vi "Module Loop.vi"(8 "error in (no error)":errorcluster, 11 "GenericGuiAO in":refnum<class "GenericGuiDO.lvclass">) -> (0 "error out":errorcluster, 3 "GenericGuiAO out":refnum<class "GenericGuiDO.lvclass">)   [LabVIEW 2020, in "VolatusDAQGenericGUI.lvlib" / "GenericGuiDO.lvclass"]
uses:
  GenericGuiDO.lvclass
  C:/dev/lv20CE/relink/lv-volatus/Volatus/Module/Module.lvclass
  Volatus/Module/Module.lvclass/Module.ctl
  Volatus/MessageQ/MessageQ.lvclass/MessageQ.ctl
  Volatus/Module/Module.lvclass
  GenericGuiDO.lvclass/GenericGuiDO.ctl
  <vilib>/Utility/error.llb/Error Cluster From Error Code.vi
  Volatus/MessageQ/MessageQ.lvclass
  VolatusDAQGenericGUI.lvlib
  C:/dev/lv20CE/relink/lv-volatus/VolatusDAQGenericGUI/GenericGuiDO/GenericGuiDO.lvclass
  Volatus/VolatusAPI/VolatusAPI.lvclass
panel:
  in  "Tree":string(tree)
  out "Cover":string="\n\n\n\n\n\n\nSelect Channel to command"
  in  "Value":bool
  out "Channel":string
  in  "Send Command":bool
  in  "Live Command":bool
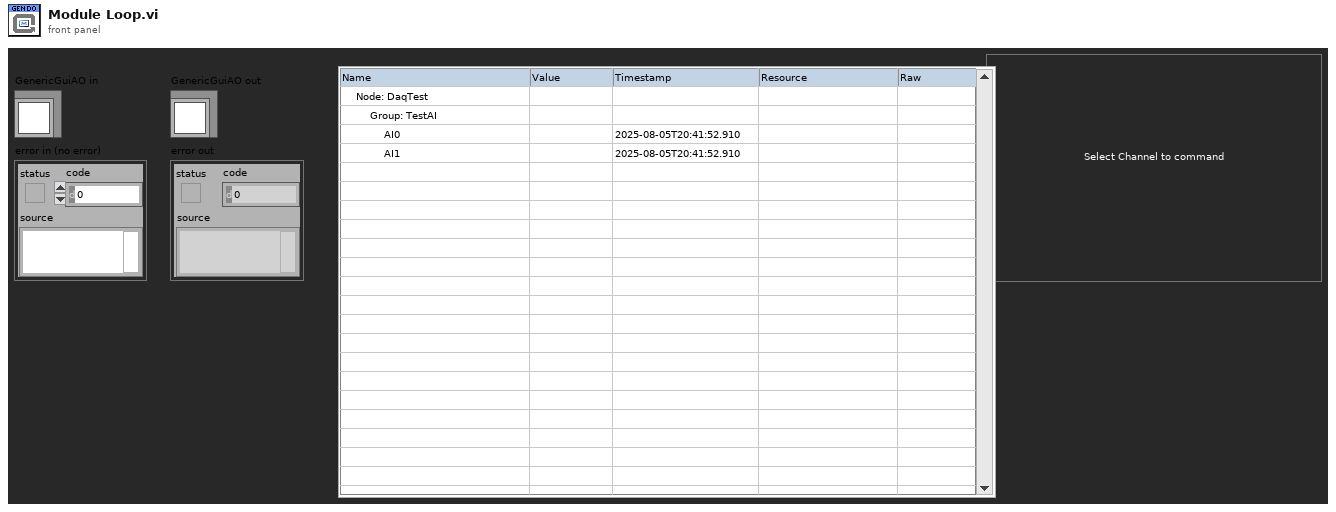
[diagram p1: front panel]
types:
  T1 = enum32{"Invalid", "Standard", "Closed", "Hidden", "Minimized", "Maximized"}
  T2 = typedef "VolatusDAQGenericGUI.lvlib/Group Info.ctl" = cluster{"Group":refnum<class "Group.lvclass">, "Channel Names":string[], "Resources":string[], "Node":string, "Task":string}
  T3 = enum8{"Enabled", "Disabled", "Disabled and Grayed Out"}
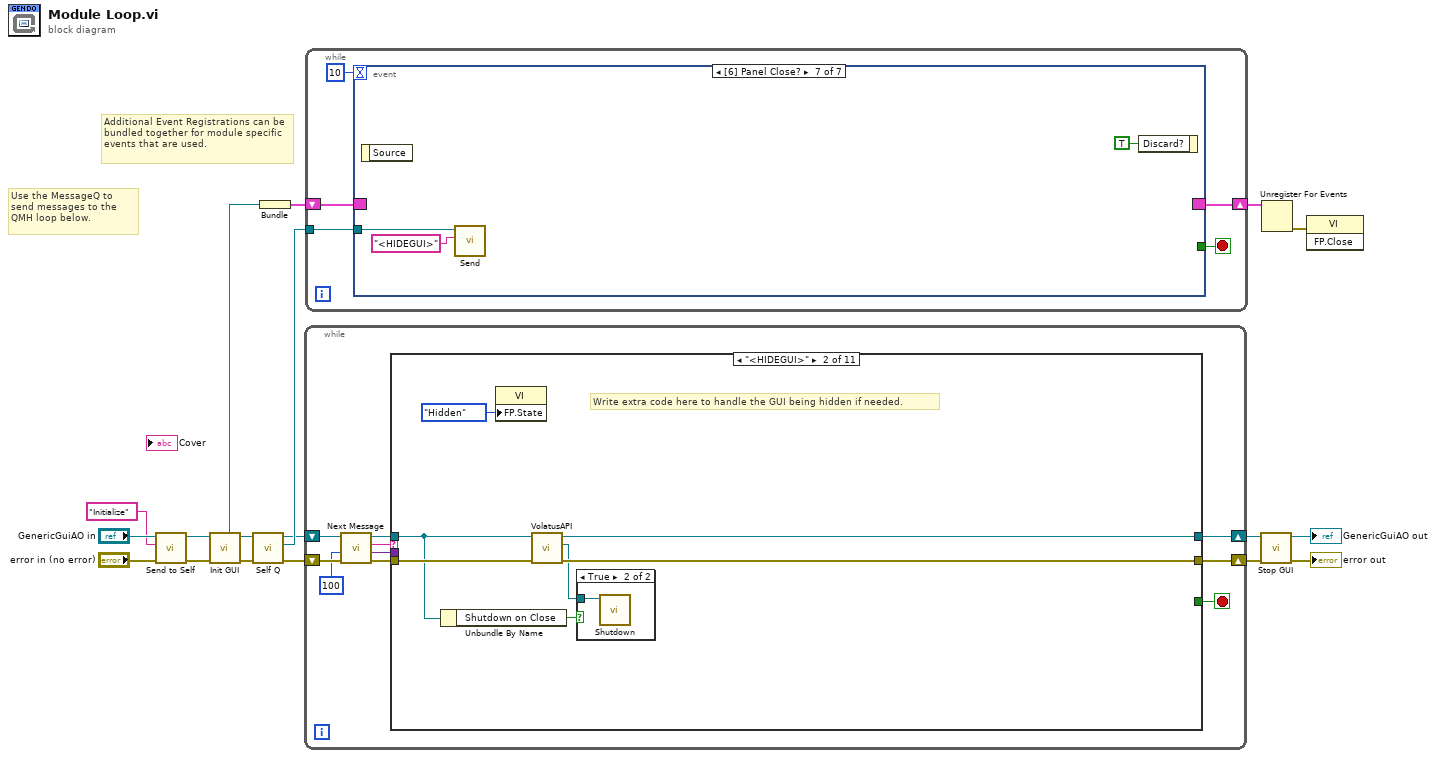
[diagram p0: block diagram]
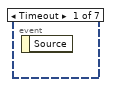
[diagram p2: hidden frame]
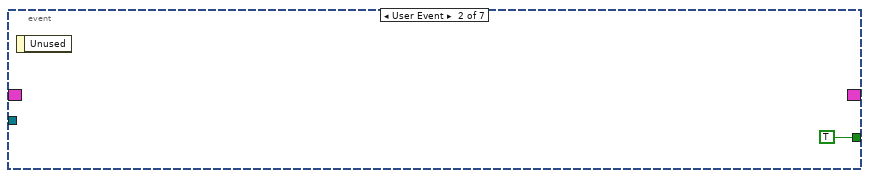
[diagram p3: hidden frame]
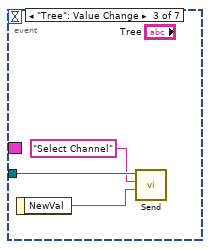
[diagram p4: hidden frame]
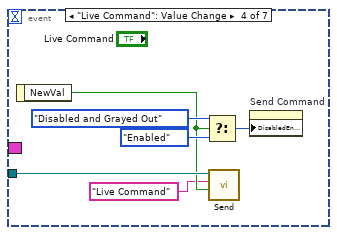
[diagram p5: hidden frame]
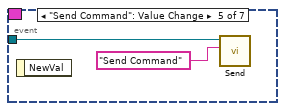
[diagram p6: hidden frame]
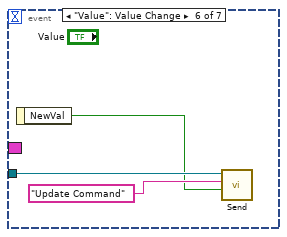
[diagram p7: hidden frame]
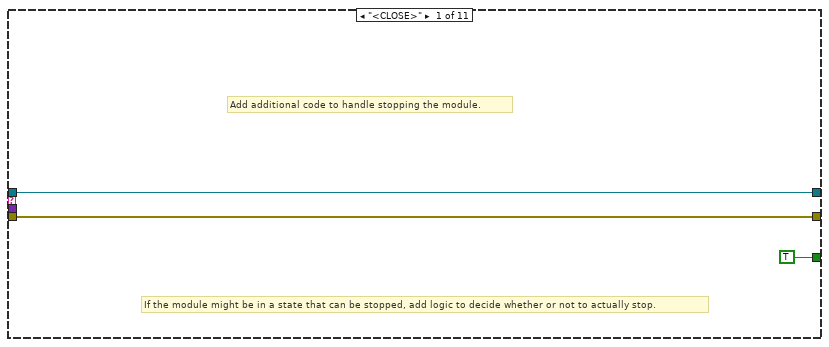
[diagram p8: hidden frame]
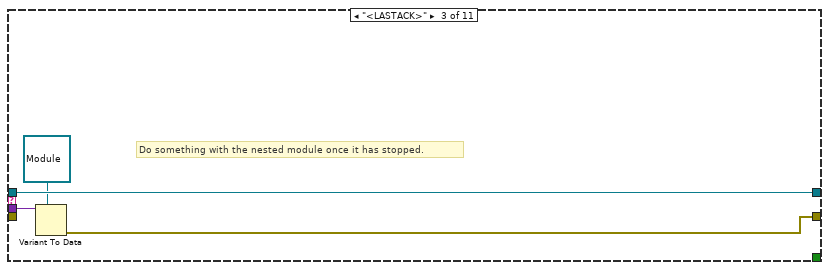
[diagram p10: hidden frame]
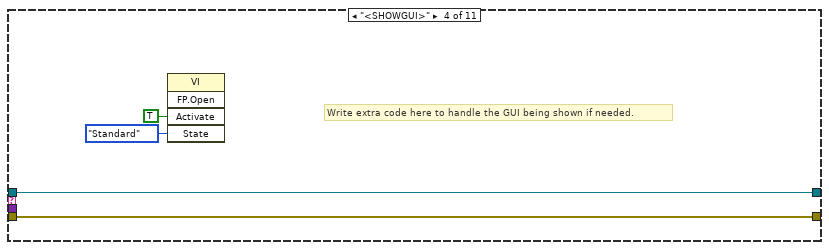
[diagram p11: hidden frame]
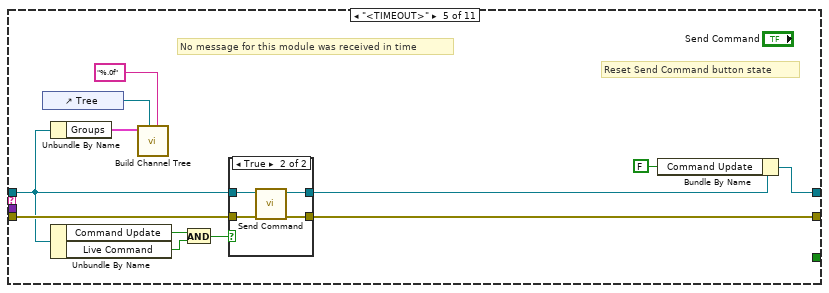
[diagram p12: hidden frame]
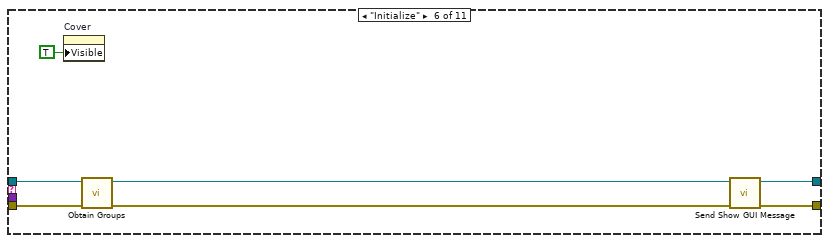
[diagram p14: hidden frame]
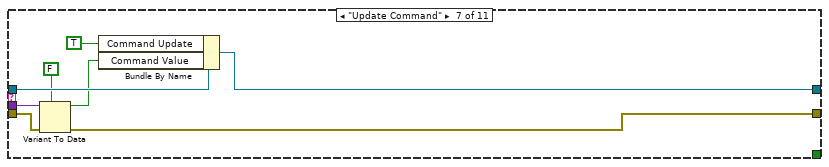
[diagram p15: hidden frame]
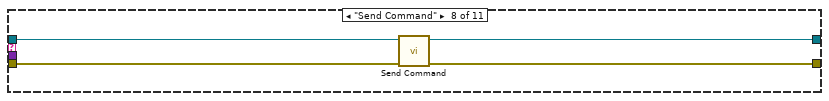
[diagram p16: hidden frame]
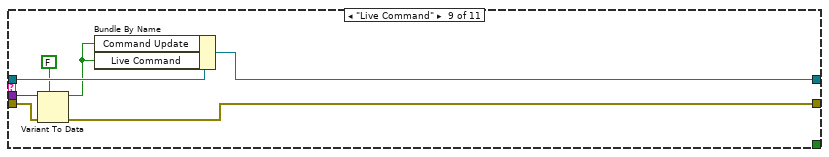
[diagram p17: hidden frame]
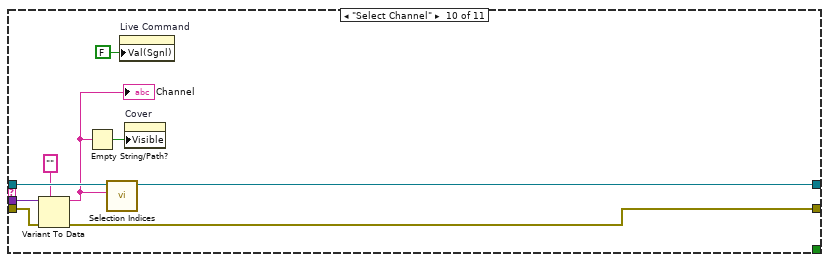
[diagram p18: hidden frame]
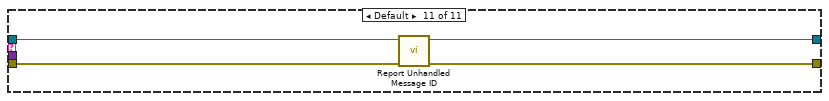
[diagram p19: hidden frame]
diagram:
  # "Additional Event Registrations can be bundled together for module specific events that are used."
  # "Use the MessageQ to send messages to the QMH loop below."
  n1 = call "Send to Self.vi"("error in (no error)"="error in (no error)", "Message ID"="Initialize", "Module in"="GenericGuiAO in") -> ("error out"=w6:errorcluster, "Module out"=w4:refnum<class "GenericGuiDO.lvclass">)  [unwired: 7 in]
  n2 = call "Init GUI.vi"("Module in"=w4) -> ("Module out"=w10:refnum<class "GenericGuiDO.lvclass">, "Event Reg"=w15:refnum<event-registration>)  [unwired: 9 in]
  n3 = call "Self Q.vi"("Module in"=w10) -> ("Self Q"=w9:refnum<class "MessageQ.lvclass">, "Module out"=w8:refnum<class "GenericGuiDO.lvclass">)  [unwired: 9 in]
  n4 = Bundle("Event Reg"=w15) -> (w11:cluster{"Event Reg":refnum<event-registration>})  [unwired: 1 in]
  n5 = while {
    shift-right: [w21] -> w13
    shift-left: w8 -> [w26]
    shift-right: [w20] -> w14
    shift-left: w6 -> [w25]
    stop <- w19 stop-if-true
    n6 = call "Next Message.vi"("error in (no error)"=w25, "Timeout ms (-1)"=100, "Module in"=w26) -> ("error out"=w24:errorcluster, "Data"=w18:variant, "ID"=w23:string, "Module out"=w22:refnum<class "GenericGuiDO.lvclass">)  [unwired: 5 in]
    n7 = case shown="\"<HIDEGUI>\"" w23 {
      tunnel: w24 -> [w27 w35 _ w43 w56 w69 w76 w81 w87 w96 w101]
      tunnel: w22 -> [w28 w30 w40 w44 w48 w67 w77 w79 w88 w97 w99]
      tunnel: [w28 w31 w40 w44 w53 w64 w72 w78 w83 w90 w98] -> w21
      tunnel: [w27 w35 w37 w43 w49 w66 w75 w80 w86 w95 w100] -> w20
      tunnel: [TRUE _ _ _ _ _ _ _ _ _ _] -> w19
      tunnel: w18 -> [_ _ w39 _ _ _ w74 _ w85 w94 _]
      frame "<CLOSE>" {
        # "If the module might be in a state that can be stopped, add logic to decide whether or not to actually stop."
        # "Add additional code to handle stopping the module."
      }
      frame "<HIDEGUI>" {
        # "Write extra code here to handle the GUI being hidden if needed."
        n8 = Unbundle By Name(w30) -> ("Shutdown on Close"=w33:bool)
        n9 = property class="VI"("FP.State"=T1."Hidden" ("Front Panel Window:State")) -> ()  [unwired: 2 in, 2 out]
        n10 = call "VolatusAPI.vi"("Module in"=w30) -> ("VolatusAPI"=w32:refnum<class "VolatusAPI.lvclass">, "Module out"=w31:refnum<class "GenericGuiDO.lvclass">)  [unwired: 9 in]
        n11 = case shown="True" w33 {
          tunnel: w32 -> [_ w36]
          frame False {
          }
          frame True {
            n12 = call "Shutdown.vi"("VolatusAPI in"=w36) -> ()  [unwired: 9 in, 2 out]
          }
        }
      }
      frame "<LASTACK>" {
        # "Do something with the nested module once it has stopped."
        n13 = Variant To Data(type=refnum<class "Module.lvclass"> refnum ("Volatus:Module"), Variant=w39) -> (error out=w37:errorcluster)  [unwired: 1 in, 1 out]
      }
      frame "<SHOWGUI>" {
        # "Write extra code here to handle the GUI being shown if needed."
        n14 = invoke class="VI" method="FP.Open"("Activate"=TRUE ("Activate?"), "State"=T1."Standard") -> ()  [unwired: 3 in, 5 out]
      }
      frame "<TIMEOUT>" {
        # "Reset Send Command button state"
        # "No message for this module was received in time"
        n15 = control-ref of="Tree"() -> (w54:refnum<vi>)
        n16 = Unbundle By Name(w48) -> ("Groups"=w55:T2[])
        n17 = Unbundle By Name(w48) -> ("Command Update"=w51:bool, "Live Command"=w50:bool)
        n18 = call "Build Channel Tree.vi"("Value Format"="%.0f", "Tree"=w54, "Groups"=w55) -> ()  [unwired: 9 in]
        n19 = And(x=w51, y=w50) -> (x .and. y?=w46:bool)
        n20 = case shown="True" w46 {
          tunnel: w56 -> [w57 w62]
          tunnel: [w57 w61] -> w49
          tunnel: w48 -> [w58 w60]
          tunnel: [w58 w59] -> w47
          frame False {
          }
          frame True {
            n21 = call "Send Command.vi"("error in (no error)"=w62, "GenericGuiAO in"=w60) -> ("error out"=w61:errorcluster, "GenericGuiAO out"=w59:refnum<class "GenericGuiDO.lvclass">)  [unwired: 8 in]
          }
        }
        n22 = Bundle By Name(cluster=w47, "Command Update"=FALSE) -> (w53:refnum<class "GenericGuiDO.lvclass">)
      }
      frame "Initialize" {
        n23 = property on="Cover" class="Str"("Visible"=TRUE) -> ()  [unwired: 2 in, 2 out]
        n24 = call "Obtain Groups.vi"("error in (no error)"=w69, "GenericGuiAO in"=w67) -> ("error out"=w68:errorcluster, "GenericGuiAO out"=w65:refnum<class "GenericGuiDO.lvclass">)  [unwired: 8 in]
        n25 = call "Send Show GUI Message.vi"("error in (no error)"=w68, "Module in"=w65) -> ("error out"=w66:errorcluster, "Module out"=w64:refnum<class "GenericGuiDO.lvclass">)  [unwired: 8 in]
      }
      frame "Update Command" {
        n26 = Variant To Data(error in=w76, type=FALSE, Variant=w74) -> (data=w71:bool, error out=w75:errorcluster)
        n27 = Bundle By Name(cluster=w77, "Command Update"=TRUE, "Command Value"=w71) -> (w72:refnum<class "GenericGuiDO.lvclass">)
      }
      frame "Send Command" {
        n28 = call "Send Command.vi"("error in (no error)"=w81, "GenericGuiAO in"=w79) -> ("error out"=w80:errorcluster, "GenericGuiAO out"=w78:refnum<class "GenericGuiDO.lvclass">)  [unwired: 8 in]
      }
      frame "Live Command" {
        n29 = Variant To Data(error in=w87, type=FALSE, Variant=w85) -> (data=w82:bool, error out=w86:errorcluster)
        n30 = Bundle By Name(cluster=w88, "Command Update"=w82, "Live Command"=w82) -> (w83:refnum<class "GenericGuiDO.lvclass">)
      }
      frame "Select Channel" {
        n31 = Variant To Data(error in=w96, type="", Variant=w94) -> (data=w89:string, error out=w95:errorcluster)
        "Channel" <- w89
        n32 = Empty String/Path?(string/path=w89) -> (empty?=w92:bool)
        n33 = call "Selection Indices.vi"("Channel Tree Tag"=w89, "GenericGuiAO in"=w97) -> ("GenericGuiAO out"=w90:refnum<class "GenericGuiDO.lvclass">)  [unwired: 8 in, 1 out]
        n34 = property on="Live Command" class="Bool (strict)"("Val(Sgnl)"=FALSE ("Value (Signaling)")) -> ()  [unwired: 2 in, 2 out]
        n35 = property on="Cover" class="Str"("Visible"=w92) -> ()  [unwired: 2 in, 2 out]
      }
      frame Default {
        n36 = call "Report Unhandled Message ID.vi"("error in (no error)"=w101, "Module in"=w99) -> ("error out"=w100:errorcluster, "Module out"=w98:refnum<class "GenericGuiDO.lvclass">)  [unwired: 8 in]
      }
    }
  }
  n37 = while {
    tunnel: w9 -> [w106]
    shift-right: [w104] -> w12
    shift-left: w11 -> [w105]
    stop <- w103 stop-if-true
    n38 = event shown="[6] Panel Close?" {
      selector: w105 -> [_ _ _ _ _ _ _]
      dyn-events: [_ _ _ _ _ _ _] -> w104
      timeout: 10 -> [_ _ _ _ _ _ _]
      tunnel: w106 -> [_ _ w110 w113 w118 w121 w123]
      tunnel: [_ TRUE _ _ _ _ _] -> w103
      event Timeout {
        n39 = event-data() -> ()  [unwired: 1 in, 1 out]
      }
      event User Event {
        n40 = event-data() -> ()  [unwired: 1 in, 1 out]
      }
      event "Tree": Value Change {
        n41 = event-data() -> ("NewVal"=w109:string)  [unwired: 1 in]
        n42 = call "Send.vi"("Data"=w109, "ID"="Select Channel", "MessageQ in"=w110) -> ()  [unwired: 7 in, 2 out]
      }
      event "Live Command": Value Change {
        n43 = event-data() -> ("NewVal"=w112:bool)  [unwired: 1 in]
        n44 = Select(t=T3."Disabled and Grayed Out" ("Disabled"), s=w112, f=T3."Enabled" ("Disabled")) -> (s? t:f=w114:T3)
        n45 = call "Send.vi"("Data"=w112, "ID"="Live Command", "MessageQ in"=w113) -> ()  [unwired: 7 in, 2 out]
        n46 = property on="Send Command" class="Bool"("DisabledEnum"=w114) -> ()  [unwired: 2 in, 2 out]
      }
      event "Send Command": Value Change {
        n47 = event-data() -> ()  [unwired: 1 in, 1 out]
        n48 = call "Send.vi"("ID"="Send Command", "MessageQ in"=w118) -> ()  [unwired: 8 in, 2 out]
      }
      event "Value": Value Change {
        n49 = event-data() -> ("NewVal"=w119:bool)  [unwired: 1 in]
        n50 = call "Send.vi"("Data"=w119, "ID"="Update Command", "MessageQ in"=w121) -> ()  [unwired: 7 in, 2 out]
      }
      event Panel Close? {
        n51 = event-data() -> ()  [unwired: 1 in, 1 out]
        n52 = call "Send.vi"("ID"="<HIDEGUI>", "MessageQ in"=w123) -> ()  [unwired: 8 in, 2 out]
        n53 = event-data("Discard?"=TRUE) -> ()  [unwired: 1 in, 1 out]
      }
    }
  }
  n54 = call "Stop GUI.vi"("error in (no error)"=w14, "Module in"=w13) -> ("error out"=→"error out":errorcluster, "Module out"=→"GenericGuiAO out":refnum<class "GenericGuiDO.lvclass">)  [unwired: 8 in]
  n55 = Unregister For Events(event registration refnum=w12) -> (error out=w16:errorcluster)  [unwired: 1 in]
  n56 = invoke class="VI" method="FP.Close"(error in=w16) -> ()  [unwired: 2 in, 3 out]
